vi "Unprocess Array Elements V2.vi"(0 "Queue In":refnum<queue>, 1 "Value":string, 2 "Read/Write Options":T2, 3 "Format String (%#_13g)":string="%#_13g", 5 "Array Variant":variant, 7 "Name In":string, 9 "Str to INI in":variant, 11 "Error In":errorcluster, 12 "Use Specified?":bool, 13 "State In":T1={"StrToSpecifiedText"=variant, "Specified Data"=variant, "Options"={"TimeStamp Format"="", "Integer format"=""}, "FloatFormat"="%#_13g"}) -> (4 "Queue Out":refnum<queue>, 8 "Data Out":string, 10 "Str to INI out":variant, 14 "State Out":T1={"StrToSpecifiedText"=variant, "Specified Data"=variant, "Options"={"TimeStamp Format"="", "Integer format"=""}, "FloatFormat"="%#_13g"}, 15 "Error Out":errorcluster)   [LabVIEW 2020]
doc: "This VI was created for use with the Read/Write Cluster VIs. It finds any array elements that have been written to file and places their value in the array.\n\nFreeware from Moore Good Ideas, www.mooregoodideas.com. Do not remove this line."
uses:
  Read Write Tag Lookup Cluster.ctl
  Read Write Options Cluster.ctl
  <vilib>/Utility/VariantDataType/VariantType.lvlib
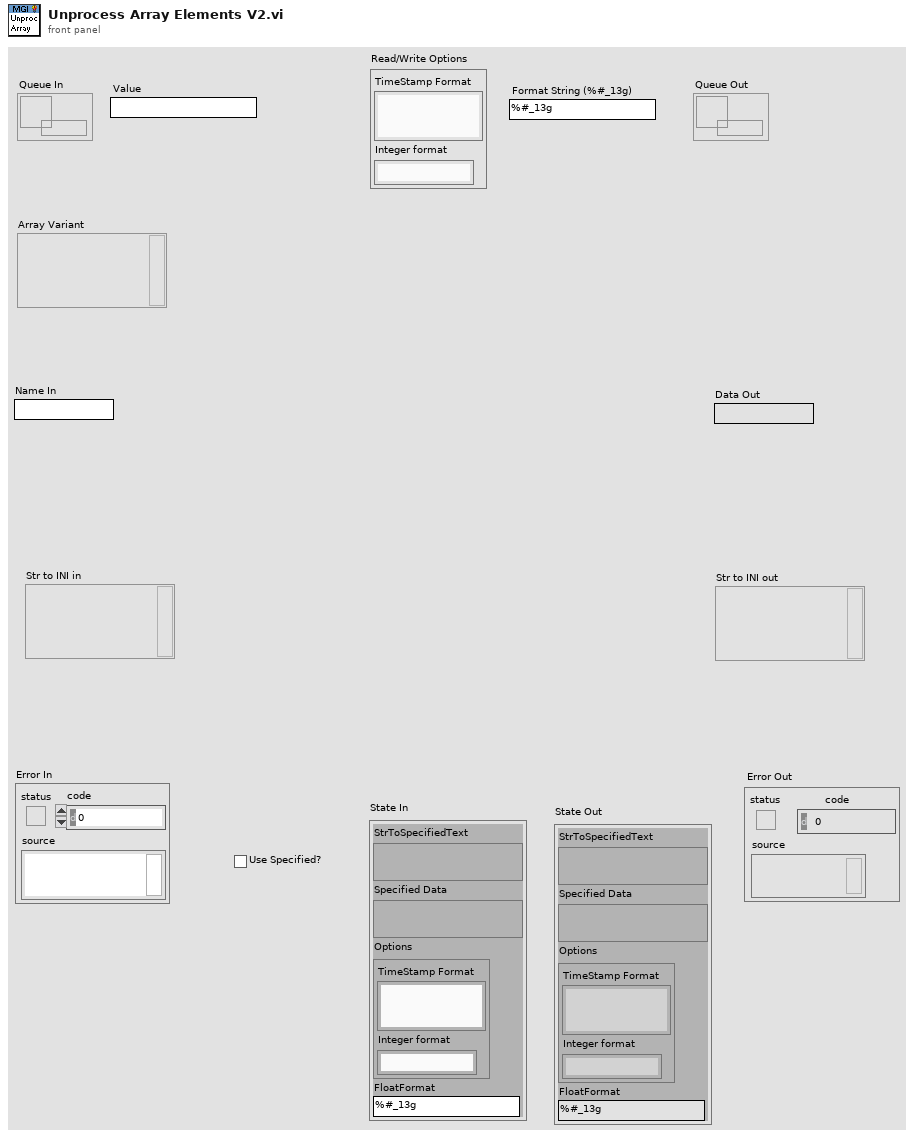
[diagram p1: front panel]
types:
  T1 = typedef "Read Write Tag Lookup Cluster.ctl" = cluster{"StrToSpecifiedText":variant, "Specified Data":variant, "Options":T2, "FloatFormat":string}
  T2 = typedef "Read Write Options Cluster.ctl" = cluster{"TimeStamp Format":string, "Integer format":string}
  T3 = typedef "VariantType.lvlib/Type.ctl" = enum8{"Invalid Type", "Void", "I8", "I16", "I32", "I64", "U8", "U16", "U32", "U64", "Single Float", "Double Float", "Extended Float", "Single Complex", "Double Complex", "Extended Complex", "Enum U8", "Enum U16", "Enum U32", "Enum U64", "Single Float With Unit", "Double Float With Unit", "Extended Float With Unit", "Single Complex with Unit", "Double Complex with Unit", "Extended Complex with Unit", "Boolean", "String", "Path", "Picture", "Tag", "Array", "Cluster", "Variant", "LV Variant", "Waveform", "Timestamp", "Digital Waveform", "Digital Data", "ExpressData", "Refnum", "External Data", "VI", "Poly VI", "LabVIEW Class Instance", "Fixed Point"}
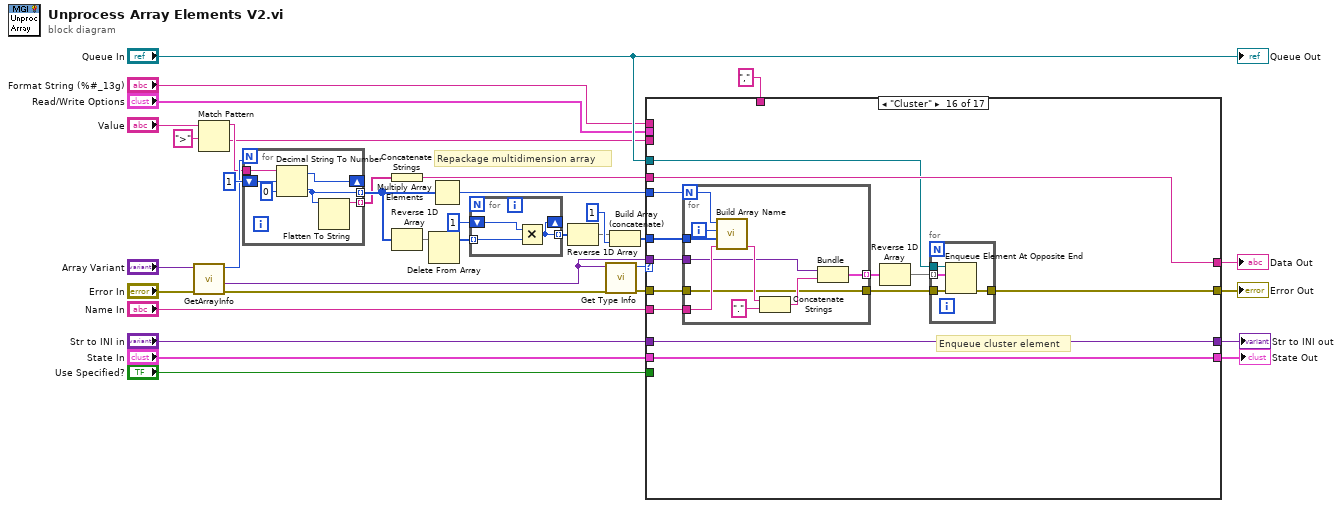
[diagram p0: block diagram]
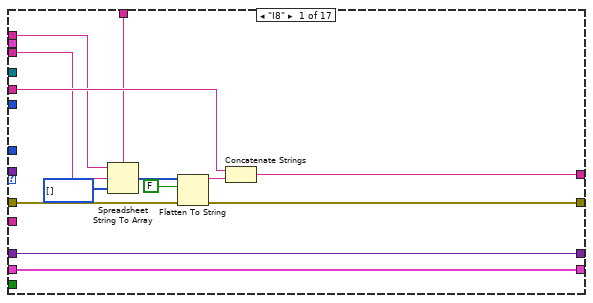
[diagram p2: hidden frame]
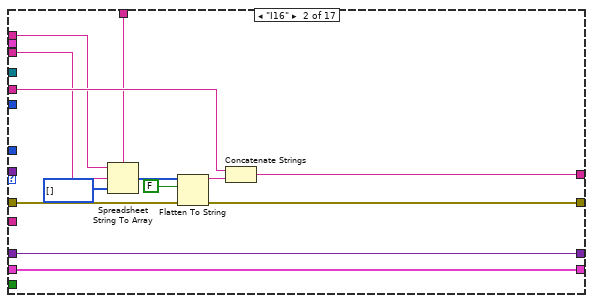
[diagram p3: hidden frame]
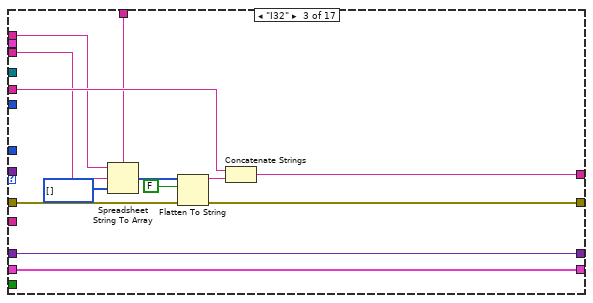
[diagram p4: hidden frame]
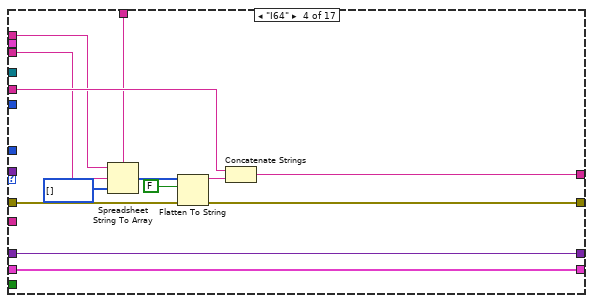
[diagram p5: hidden frame]
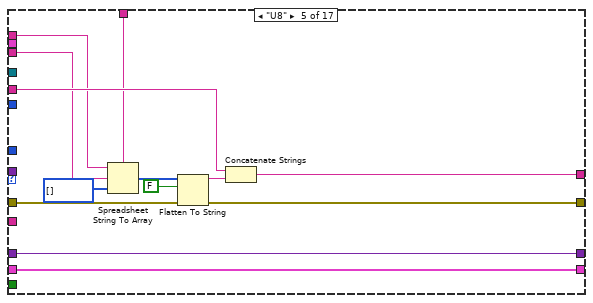
[diagram p6: hidden frame]
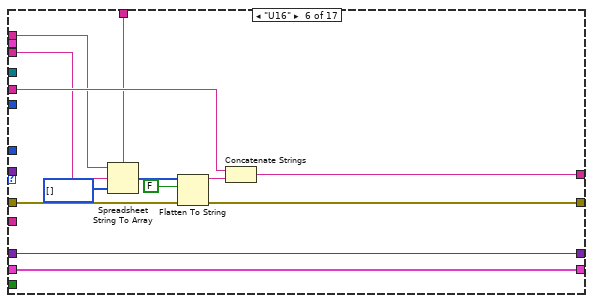
[diagram p7: hidden frame]
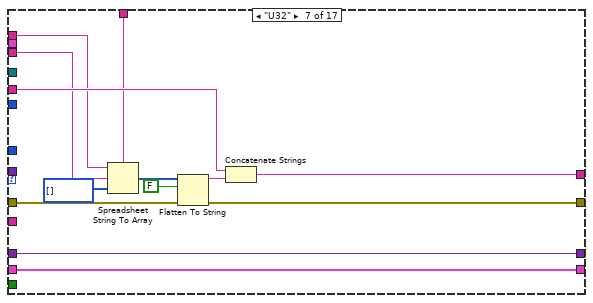
[diagram p8: hidden frame]
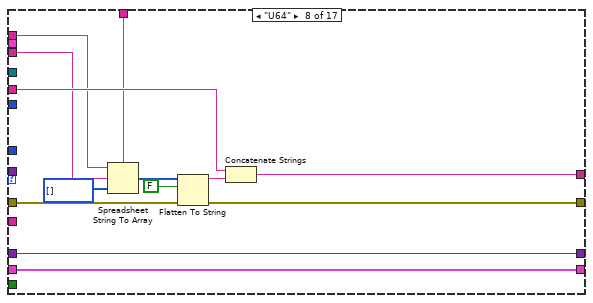
[diagram p9: hidden frame]
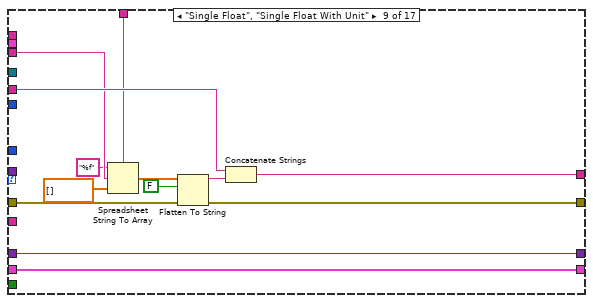
[diagram p10: hidden frame]
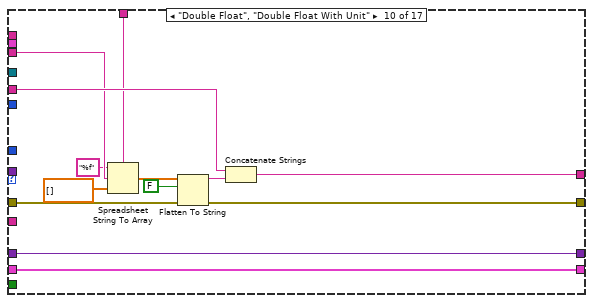
[diagram p11: hidden frame]
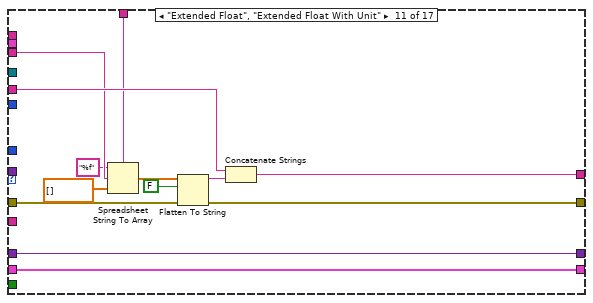
[diagram p12: hidden frame]
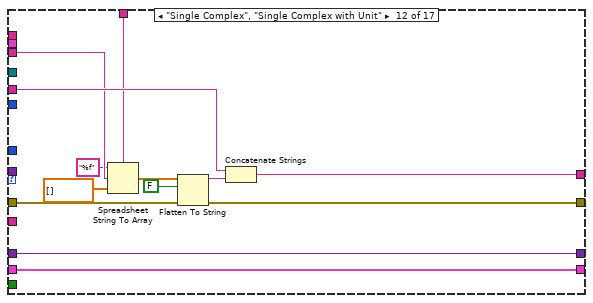
[diagram p13: hidden frame]
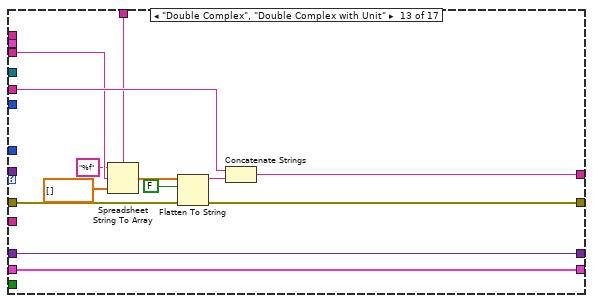
[diagram p14: hidden frame]
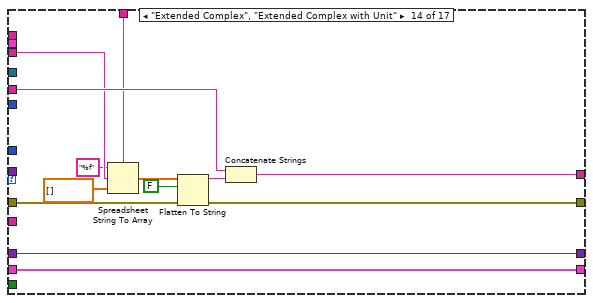
[diagram p15: hidden frame]
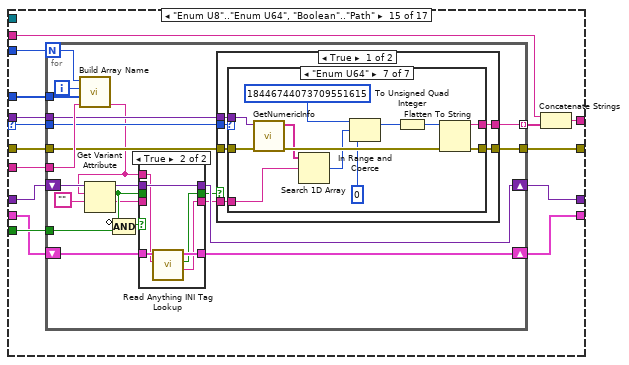
[diagram p16: hidden frame]
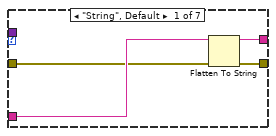
[diagram p18: hidden frame]
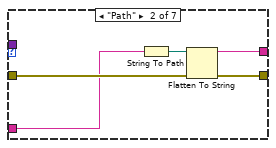
[diagram p19: hidden frame]
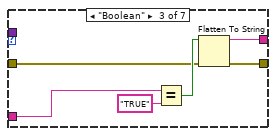
[diagram p20: hidden frame]
diagram:
  # "Repackage multidimension array"
  n1 = call <vilib>:"GetArrayInfo.vi"("error in (no error)"="Error In", "Variant"="Array Variant") -> ("error out"=w20:errorcluster, "ArrayElement"=w21:variant, "NDims"=w18:i32)  [unwired: 6 in, 1 out]
  n2 = Match Pattern(string="Value", regular expression=">") -> (before substring=w11:string, after substring=w10:string)  [unwired: 1 in, 2 out]
  n3 = for {
    N: w18 -> [_]
    shift-right: [w40] -> _
    shift-left: 1 ("offset past number") -> [w39]
    tunnel: w11 -> [w41]
    tunnel: [w37] -> w17 mode=indexing
    tunnel: [w36] -> w16 mode=indexing
    n4 = Decimal String To Number(string=w41, offset=w39, default (0L)=u32 0 ("default (0 I32)")) -> (offset past number=w40:i32, number=w37:u32)
    n5 = Flatten To String(anything=w37) -> (data string=w36:string)  [unwired: 3 in, 2 out]
  }
  n6 = Concatenate Strings(w16) -> (w15:string)
  n7 = Reverse 1D Array(array=w17) -> (reversed array=w25:u32[])
  n8 = Delete From Array(array=w25) -> (array with subset deleted=w26:u32[])  [unwired: 2 in, 1 out]
  n9 = Multiply Array Elements(1:w17) -> (0:w32:u32)
  n10 = for {
    tunnel: w26 -> [w44] mode=indexing
    shift-right: [w42] -> _
    shift-left: i8 1 -> [w43]
    tunnel: [w42] -> w28 mode=indexing
    n11 = Multiply(x=w43, y=w44) -> (x*y=w42:u32)
  }
  n12 = Reverse 1D Array(array=w28) -> (reversed array=w29:u32[])
  n13 = call "Get Type Info.vi"("Error In"=w20, "Variant"=w21) -> ("Error Out"=w33:errorcluster, "Type Enum"=w9:T3)  [unwired: 7 in, 1 out]
  n14 = Build Array (concatenate)(w29, i8 1) -> (w24:u32[])
  n15 = case shown="\"Cluster\"" w9 {
    selector: w9 -> [_ _ _ _ _ _ _ _ _ _ _ _ _ _ w227 _ _]
    tunnel: [w57 w70 w83 w96 w109 w122 w135 w148 w161 w174 w187 w200 w213 w226 w241 w380 w414] -> w23
    tunnel: w33 -> [w56 w69 w82 w95 w108 w121 w134 w147 w160 w173 w186 w199 w212 w225 w240 w387 w414]
    tunnel: w15 -> [w54 w67 w80 w93 w106 w119 w132 w145 w158 w171 w184 w197 w210 w223 w234 w383 w412]
    tunnel: w32 -> [_ _ _ _ _ _ _ _ _ _ _ _ _ _ w239 w386 _]
    tunnel: "Name In" -> [_ _ _ _ _ _ _ _ _ _ _ _ _ _ w238 w385 _]
    tunnel: w24 -> [_ _ _ _ _ _ _ _ _ _ _ _ _ _ w237 w384 _]
    tunnel: "Queue In" -> [_ _ _ _ _ _ _ _ _ _ _ _ _ _ _ w379 _]
    tunnel: w21 -> [_ _ _ _ _ _ _ _ _ _ _ _ _ _ w232 w382 _]
    tunnel: "Str to INI in" -> [w46 w59 w72 w85 w98 w111 w124 w137 w150 w163 w176 w189 w202 w215 w236 w376 w403]
    tunnel: [w55 w68 w81 w94 w107 w120 w133 w146 w159 w172 w185 w198 w211 w224 w233 w383 w411] -> w14
    tunnel: w10 -> [w53 w66 w79 w92 w105 w118 w131 w144 w157 w170 w183 w196 w209 w222 _ _ w410]
    tunnel: "," ("delimiter (Tab)") -> [w48 w61 w74 w87 w100 w113 w126 w139 w151 w164 w177 w190 w203 w216 _ _ _]
    tunnel: "Read/Write Options" -> [_ _ _ _ _ _ _ _ _ _ _ _ _ _ _ _ _]
    tunnel: "Format String (%#_13g)" -> [w47 w60 w73 w86 w99 w112 w125 w138 _ _ _ _ _ _ _ _ _]
    tunnel: [w46 w59 w72 w85 w98 w111 w124 w137 w150 w163 w176 w189 w202 w215 w231 w376 w403] -> w1
    tunnel: "State In" -> [w45 w58 w71 w84 w97 w110 w123 w136 w149 w162 w175 w188 w201 w214 w229 w375 w402]
    tunnel: "Use Specified?" -> [_ _ _ _ _ _ _ _ _ _ _ _ _ _ w230 _ _]
    tunnel: [w45 w58 w71 w84 w97 w110 w123 w136 w149 w162 w175 w188 w201 w214 w228 w375 w402] -> w2
    frame "I8" {
      n16 = Spreadsheet String To Array(delimiter (Tab)=w48, format string=w47, spreadsheet string=w53, array type (2D Dbl)=i8[] []) -> (array=w52:i8[])
      n17 = Flatten To String(anything=w52, prepend array or string size? (T)=FALSE, error in (no error)=w56) -> (data string=w49:string, error out=w57:errorcluster)  [unwired: 1 in, 1 out]
      n18 = Concatenate Strings(w54, w49) -> (w55:string)
    }
    frame "I16" {
      n19 = Spreadsheet String To Array(delimiter (Tab)=w61, format string=w60, spreadsheet string=w66, array type (2D Dbl)=i16[] []) -> (array=w65:i16[])
      n20 = Flatten To String(anything=w65, prepend array or string size? (T)=FALSE, error in (no error)=w69) -> (data string=w62:string, error out=w70:errorcluster)  [unwired: 1 in, 1 out]
      n21 = Concatenate Strings(w67, w62) -> (w68:string)
    }
    frame "I32" {
      n22 = Spreadsheet String To Array(delimiter (Tab)=w74, format string=w73, spreadsheet string=w79, array type (2D Dbl)=i32[] []) -> (array=w78:i32[])
      n23 = Flatten To String(anything=w78, prepend array or string size? (T)=FALSE, error in (no error)=w82) -> (data string=w75:string, error out=w83:errorcluster)  [unwired: 1 in, 1 out]
      n24 = Concatenate Strings(w80, w75) -> (w81:string)
    }
    frame "I64" {
      n25 = Spreadsheet String To Array(delimiter (Tab)=w87, format string=w86, spreadsheet string=w92, array type (2D Dbl)=i64[] []) -> (array=w91:i64[])
      n26 = Flatten To String(anything=w91, prepend array or string size? (T)=FALSE, error in (no error)=w95) -> (data string=w88:string, error out=w96:errorcluster)  [unwired: 1 in, 1 out]
      n27 = Concatenate Strings(w93, w88) -> (w94:string)
    }
    frame "U8" {
      n28 = Spreadsheet String To Array(delimiter (Tab)=w100, format string=w99, spreadsheet string=w105, array type (2D Dbl)=u8[] []) -> (array=w104:u8[])
      n29 = Flatten To String(anything=w104, prepend array or string size? (T)=FALSE, error in (no error)=w108) -> (data string=w101:string, error out=w109:errorcluster)  [unwired: 1 in, 1 out]
      n30 = Concatenate Strings(w106, w101) -> (w107:string)
    }
    frame "U16" {
      n31 = Spreadsheet String To Array(delimiter (Tab)=w113, format string=w112, spreadsheet string=w118, array type (2D Dbl)=u16[] []) -> (array=w117:u16[])
      n32 = Flatten To String(anything=w117, prepend array or string size? (T)=FALSE, error in (no error)=w121) -> (data string=w114:string, error out=w122:errorcluster)  [unwired: 1 in, 1 out]
      n33 = Concatenate Strings(w119, w114) -> (w120:string)
    }
    frame "U32" {
      n34 = Spreadsheet String To Array(delimiter (Tab)=w126, format string=w125, spreadsheet string=w131, array type (2D Dbl)=u32[] []) -> (array=w130:u32[])
      n35 = Flatten To String(anything=w130, prepend array or string size? (T)=FALSE, error in (no error)=w134) -> (data string=w127:string, error out=w135:errorcluster)  [unwired: 1 in, 1 out]
      n36 = Concatenate Strings(w132, w127) -> (w133:string)
    }
    frame "U64" {
      n37 = Spreadsheet String To Array(delimiter (Tab)=w139, format string=w138, spreadsheet string=w144, array type (2D Dbl)=u64[] []) -> (array=w143:u64[])
      n38 = Flatten To String(anything=w143, prepend array or string size? (T)=FALSE, error in (no error)=w147) -> (data string=w140:string, error out=w148:errorcluster)  [unwired: 1 in, 1 out]
      n39 = Concatenate Strings(w145, w140) -> (w146:string)
    }
    frame "Single Float", "Single Float With Unit" {
      n40 = Spreadsheet String To Array(delimiter (Tab)=w151, format string="%f", spreadsheet string=w157, array type (2D Dbl)=sgl[] []) -> (array=w155:sgl[])
      n41 = Flatten To String(anything=w155, prepend array or string size? (T)=FALSE, error in (no error)=w160) -> (data string=w152:string, error out=w161:errorcluster)  [unwired: 1 in, 1 out]
      n42 = Concatenate Strings(w158, w152) -> (w159:string)
    }
    frame "Double Float", "Double Float With Unit" {
      n43 = Spreadsheet String To Array(delimiter (Tab)=w164, format string="%f", spreadsheet string=w170, array type (2D Dbl)=dbl[] []) -> (array=w168:dbl[])
      n44 = Flatten To String(anything=w168, prepend array or string size? (T)=FALSE, error in (no error)=w173) -> (data string=w165:string, error out=w174:errorcluster)  [unwired: 1 in, 1 out]
      n45 = Concatenate Strings(w171, w165) -> (w172:string)
    }
    frame "Extended Float", "Extended Float With Unit" {
      n46 = Spreadsheet String To Array(delimiter (Tab)=w177, format string="%f", spreadsheet string=w183, array type (2D Dbl)=ext[] []) -> (array=w181:ext[])
      n47 = Flatten To String(anything=w181, prepend array or string size? (T)=FALSE, error in (no error)=w186) -> (data string=w178:string, error out=w187:errorcluster)  [unwired: 1 in, 1 out]
      n48 = Concatenate Strings(w184, w178) -> (w185:string)
    }
    frame "Single Complex", "Single Complex with Unit" {
      n49 = Spreadsheet String To Array(delimiter (Tab)=w190, format string="%f", spreadsheet string=w196, array type (2D Dbl)=csg[] []) -> (array=w194:csg[])
      n50 = Flatten To String(anything=w194, prepend array or string size? (T)=FALSE, error in (no error)=w199) -> (data string=w191:string, error out=w200:errorcluster)  [unwired: 1 in, 1 out]
      n51 = Concatenate Strings(w197, w191) -> (w198:string)
    }
    frame "Double Complex", "Double Complex with Unit" {
      n52 = Spreadsheet String To Array(delimiter (Tab)=w203, format string="%f", spreadsheet string=w209, array type (2D Dbl)=cdb[] []) -> (array=w207:cdb[])
      n53 = Flatten To String(anything=w207, prepend array or string size? (T)=FALSE, error in (no error)=w212) -> (data string=w204:string, error out=w213:errorcluster)  [unwired: 1 in, 1 out]
      n54 = Concatenate Strings(w210, w204) -> (w211:string)
    }
    frame "Extended Complex", "Extended Complex with Unit" {
      n55 = Spreadsheet String To Array(delimiter (Tab)=w216, format string="%f", spreadsheet string=w222, array type (2D Dbl)=cxt[] []) -> (array=w220:cxt[])
      n56 = Flatten To String(anything=w220, prepend array or string size? (T)=FALSE, error in (no error)=w225) -> (data string=w217:string, error out=w226:errorcluster)  [unwired: 1 in, 1 out]
      n57 = Concatenate Strings(w223, w217) -> (w224:string)
    }
    frame "Enum U8".."Enum U64", "Boolean".."Path" {
      n58 = for {
        N: w239 -> [w263]
        tunnel: [w258] -> w241
        tunnel: w240 -> [w259]
        tunnel: w238 -> [w260]
        tunnel: w237 -> [w261]
        tunnel: [w257] -> w235 mode=indexing
        tunnel: w232 -> [w256]
        shift-right: [w246] -> w231
        shift-left: w236 -> [w251]
        tunnel: w230 -> [w250]
        shift-right: [w247] -> w228
        shift-left: w229 -> [w248]
        tunnel: w227 -> [w243]
        i -> [w262]
        n59 = call "Build Array Name.vi"("Name In"=w260, "Array"=w261, "Iteration"=w262, "Iterations"=w263) -> ("Name Out"=w242:string)  [unwired: 7 in]
        n60 = Get Variant Attribute(Variant=w251, name=w242, default value (empty Variant)="") -> (duplicate Variant=w255:variant, found=w254:bool, value=w253:string)  [unwired: 1 in, 1 out]
        n61 = Compound Arithmetic op=AND(invert w254, w250) -> (w249:bool)
        n62 = case shown="True" w249 {
          tunnel: w253 -> [w265 _]
          tunnel: w254 -> [w266 _]
          tunnel: w242 -> [_ w268]
          tunnel: w255 -> [w267 w272]
          tunnel: [w267 w272] -> w246
          tunnel: [w266 w270] -> w245
          tunnel: [w265 w269] -> w244
          tunnel: w248 -> [w264 w273]
          tunnel: [w264 w271] -> w247
          frame False {
          }
          frame True {
            n63 = call "Read Anything INI Tag Lookup.vi"("Str"=w268, "State In"=w273) -> ("INI Text"=w269:string, "Text Found?"=w270:bool, "State Out"=w271:T1)  [unwired: 7 in]
          }
        }
        n64 = case shown="True" w245 {
          tunnel: [w278 w344] -> w258
          tunnel: w259 -> [w277 w345]
          tunnel: [w279 w346] -> w257
          tunnel: w256 -> [w276 _]
          tunnel: w244 -> [w275 _]
          tunnel: w243 -> [w274 w343]
          frame True {
            n65 = case shown="\"Enum U64\"" w274 {
              tunnel: [w280 w285 w290 w306 w318 w330 w342] -> w279
              tunnel: [w281 w286 w289 w305 w317 w329 w341] -> w278
              tunnel: w277 -> [w282 w287 w292 w304 w316 w328 w340]
              tunnel: w276 -> [_ _ _ w303 w315 w327 w339]
              tunnel: w275 -> [w283 w284 w291 w299 w311 w323 w335]
              frame "String", Default {
                n66 = Flatten To String(anything=w283, error in (no error)=w282) -> (data string=w280:string, error out=w281:errorcluster)  [unwired: 2 in, 1 out]
              }
              frame "Path" {
                n67 = String To Path(string=w284) -> (path=w288:path)
                n68 = Flatten To String(anything=w288, error in (no error)=w287) -> (data string=w285:string, error out=w286:errorcluster)  [unwired: 2 in, 1 out]
              }
              frame "Boolean" {
                n69 = Equal?(x=w291, y="TRUE") -> (x = y?=w293:bool)
                n70 = Flatten To String(anything=w293, error in (no error)=w292) -> (data string=w290:string, error out=w289:errorcluster)  [unwired: 2 in, 1 out]
              }
              frame "Enum U8" {
                n71 = call <vilib>:"GetNumericInfo.vi"("error in (no error)"=w304, "Variant"=w303) -> ("error out"=w302:errorcluster, "EnumNames"=w300:string[])  [unwired: 6 in, 2 out]
                n72 = Search 1D Array(1D array=w300, element=w299) -> (index of element=w301:i32)  [unwired: 1 in]
                n73 = In Range and Coerce(upper limit=255, x=w301, lower limit=0) -> (coerced(x)=w298:i32)  [unwired: 1 out]
                n74 = To Unsigned Byte Integer(number=w298) -> (unsigned 8bit integer=w297:u8)
                n75 = Flatten To String(anything=w297, error in (no error)=w302) -> (data string=w306:string, error out=w305:errorcluster)  [unwired: 2 in, 1 out]
              }
              frame "Enum U16" {
                n76 = call <vilib>:"GetNumericInfo.vi"("error in (no error)"=w316, "Variant"=w315) -> ("error out"=w314:errorcluster, "EnumNames"=w312:string[])  [unwired: 6 in, 2 out]
                n77 = Search 1D Array(1D array=w312, element=w311) -> (index of element=w313:i32)  [unwired: 1 in]
                n78 = In Range and Coerce(upper limit=65535, x=w313, lower limit=0) -> (coerced(x)=w310:i32)  [unwired: 1 out]
                n79 = To Unsigned Word Integer(number=w310) -> (unsigned 16bit integer=w309:u16)
                n80 = Flatten To String(anything=w309, error in (no error)=w314) -> (data string=w318:string, error out=w317:errorcluster)  [unwired: 2 in, 1 out]
              }
              frame "Enum U32" {
                n81 = call <vilib>:"GetNumericInfo.vi"("error in (no error)"=w328, "Variant"=w327) -> ("error out"=w326:errorcluster, "EnumNames"=w324:string[])  [unwired: 6 in, 2 out]
                n82 = Search 1D Array(1D array=w324, element=w323) -> (index of element=w325:i32)  [unwired: 1 in]
                n83 = In Range and Coerce(upper limit=u32 4294967295, x=w325, lower limit=0) -> (coerced(x)=w322:u32)  [unwired: 1 out]
                n84 = To Unsigned Long Integer(number=w322) -> (unsigned 32bit integer=w321:u32)
                n85 = Flatten To String(anything=w321, error in (no error)=w326) -> (data string=w330:string, error out=w329:errorcluster)  [unwired: 2 in, 1 out]
              }
              frame "Enum U64" {
                n86 = call <vilib>:"GetNumericInfo.vi"("error in (no error)"=w340, "Variant"=w339) -> ("error out"=w338:errorcluster, "EnumNames"=w336:string[])  [unwired: 6 in, 2 out]
                n87 = Search 1D Array(1D array=w336, element=w335) -> (index of element=w337:i32)  [unwired: 1 in]
                n88 = In Range and Coerce(upper limit=u64 18446744073709551615, x=w337, lower limit=0) -> (coerced(x)=w333:u64)  [unwired: 1 out]
                n89 = To Unsigned Quad Integer(1:w333) -> (0:w332:u64)
                n90 = Flatten To String(anything=w332, error in (no error)=w338) -> (data string=w342:string, error out=w341:errorcluster)  [unwired: 2 in, 1 out]
              }
            }
          }
          frame False {
            n91 = case shown="\"Enum U64\"" w343 {
              tunnel: [w347 w353 w355 w362 w366 w370 w374] -> w346
              tunnel: w345 -> [w349 w351 w357 w360 w364 w368 w372]
              tunnel: [w348 w352 w356 w359 w363 w367 w371] -> w344
              frame "String", Default {
                n92 = Flatten To String(anything="", error in (no error)=w349) -> (data string=w347:string, error out=w348:errorcluster)  [unwired: 2 in, 1 out]
              }
              frame "Path" {
                n93 = Flatten To String(anything=path "", error in (no error)=w351) -> (data string=w353:string, error out=w352:errorcluster)  [unwired: 2 in, 1 out]
              }
              frame "Boolean" {
                n94 = Flatten To String(anything=FALSE, error in (no error)=w357) -> (data string=w355:string, error out=w356:errorcluster)  [unwired: 2 in, 1 out]
              }
              frame "Enum U8" {
                n95 = Flatten To String(anything=u8 0, error in (no error)=w360) -> (data string=w362:string, error out=w359:errorcluster)  [unwired: 2 in, 1 out]
              }
              frame "Enum U16" {
                n96 = Flatten To String(anything=u16 0, error in (no error)=w364) -> (data string=w366:string, error out=w363:errorcluster)  [unwired: 2 in, 1 out]
              }
              frame "Enum U32" {
                n97 = Flatten To String(anything=u32 0, error in (no error)=w368) -> (data string=w370:string, error out=w367:errorcluster)  [unwired: 2 in, 1 out]
              }
              frame "Enum U64" {
                n98 = Flatten To String(anything=u64 0, error in (no error)=w372) -> (data string=w374:string, error out=w371:errorcluster)  [unwired: 2 in, 1 out]
              }
            }
          }
        }
      }
      n99 = Concatenate Strings(w234, w235) -> (w233:string)
    }
    frame "Cluster" {
      # "Enqueue cluster element"
      n100 = for {
        N: w386 -> [w401]
        tunnel: w387 -> [w393]
        tunnel: w385 -> [w398]
        tunnel: w384 -> [w399]
        tunnel: w382 -> [w394]
        tunnel: [w393] -> w381
        tunnel: [w392] -> w378 mode=indexing
        i -> [w400]
        n101 = call "Build Array Name.vi"("Name In"=w398, "Array"=w399, "Iteration"=w400, "Iterations"=w401) -> ("Name Out"=w395:string)  [unwired: 7 in]
        n102 = Concatenate Strings(w395, "." ("string")) -> (w397:string)
        n103 = Bundle("ArrayElement"=w394, w397) -> (w392:cluster{"ArrayElement":variant, string})  [unwired: 1 in]
      }
      n104 = Reverse 1D Array(array=w378) -> (reversed array=w377:cluster{"ArrayElement":variant, string}[])
      n105 = for {
        tunnel: w381 -> [w391]
        tunnel: [w390] -> w380
        tunnel: w379 -> [w389]
        tunnel: w377 -> [w388] mode=indexing
        n106 = Enqueue Element At Opposite End(queue=w389, element=w388, error in (no error)=w391) -> (error out=w390:errorcluster)  [unwired: 1 in, 2 out]
      }
    }
    frame Default {
      n107 = String Subset(string=w410, offset (0)=2) -> (substring=w407:string)  [unwired: 1 in]
      n108 = String Length(string=w407) -> (length=w408:i32)
      n109 = Multiply(x=0.5, y=w408) -> (x*y=w409:dbl)
      n110 = for {
        N: w409 -> [_]
        tunnel: w407 -> [w418]
        tunnel: [w420] -> w405 mode=indexing
        i -> [w417]
        w416 = 2 ("length (rest)")
        n111 = Multiply(x=w417, y=w416) -> (x*y=w415:i32)
        n112 = String Subset(string=w418, offset (0)=w415, length (rest)=w416) -> (substring=w419:string)
        n113 = Hexadecimal String To Number(string=w419, default (0uL)=u8 0 ("default (0 U32)")) -> (number=w420:u8)  [unwired: 1 in, 1 out]
      }
      n114 = Byte Array To String(unsigned byte array=w405) -> (string=w413:string)
      n115 = Concatenate Strings(w412, w413) -> (w411:string)
    }
  }
  "Error Out" <- w23
  "Data Out" <- w14
  "State Out" <- w2
  "Str to INI out" <- w1
  "Queue Out" <- "Queue In"
